vi "Spectrograph_getCurrentTime.vi"(8 "error in (no error)":errorcluster) -> (0 "error out":errorcluster, 3 "function return":dbl)   [LabVIEW 2016, in "SALLV_Spectrograph.lvlib"]
doc: "double Spectrograph_shm_getCurrentTimeLV();"
uses:
  SALLV_Spectrograph.lvlib
  SALLV_Spectrograph.so
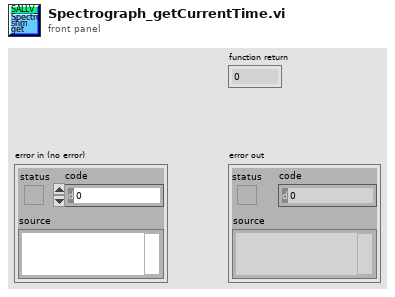
[diagram p1: front panel]
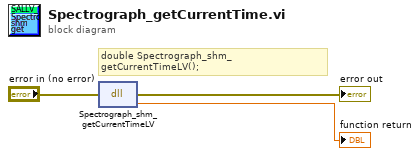
[diagram p0: block diagram]
diagram:
  # "double Spectrograph_shm_getCurrentTimeLV();"
  n1 = dll-call lib="home/harini/TCS/SALLV_Spectrograph/SALLV_Spectrograph.*" fn="Spectrograph_shm_getCurrentTimeLV"(error in="error in (no error)") -> (error out=→"error out":errorcluster, →"function return":dbl)  [unwired: 2 in, 1 out]
